vi "HOST Player Entry.vi"() -> ()   [LabVIEW 2026]
uses:
  Host State.ctl
  Leaderboard Announcement.ctl
  RT Commands.ctl
  RT Image.ctl
  Game Settings.ctl
  RT States.ctl
  Score.ctl
  SideSelector.ctl
  <vilib>/event_ctls.llb/eventvkey.ctl
  cee997e7-3729-4498-a080-51e98f020221.vi
  5b16e98e-8c62-4f4c-9228-1465c9ac843a.vi
  e3477a6d-3302-43e1-9f71-62fb47c8ca94.vi
  e2e9e0fd-3f68-41fd-9f22-0fd033314a53.vi
  <extravilib>/ChannelInstances/Tag-bool/Read With Abort.vi
  <extravilib>/ChannelInstances/Tag-bool/Write With Abort.vi
  <extravilib>/ChannelInstances/Tag-bool/Instantiate.vi
  <extravilib>/ChannelInstances/Tag-bool/EndpointRead.vi
  <extravilib>/ChannelInstances/Tag-bool/Endpoint.vi
  <extravilib>/ChannelInstances/Tag-bool.lvlib
panel:
  in  "path to PNG file":path
  in  "Button 1":bool
  in  "Player 1 Name":string
  in  "Button 2":bool
  in  "Player 2 Name":string
  in  "GO":bool
  out "error IO":errorcluster
  out "Status":string
  # "(ESC to abort round)"
  # "(Ctl+Shfit+GO! to terminate program)"
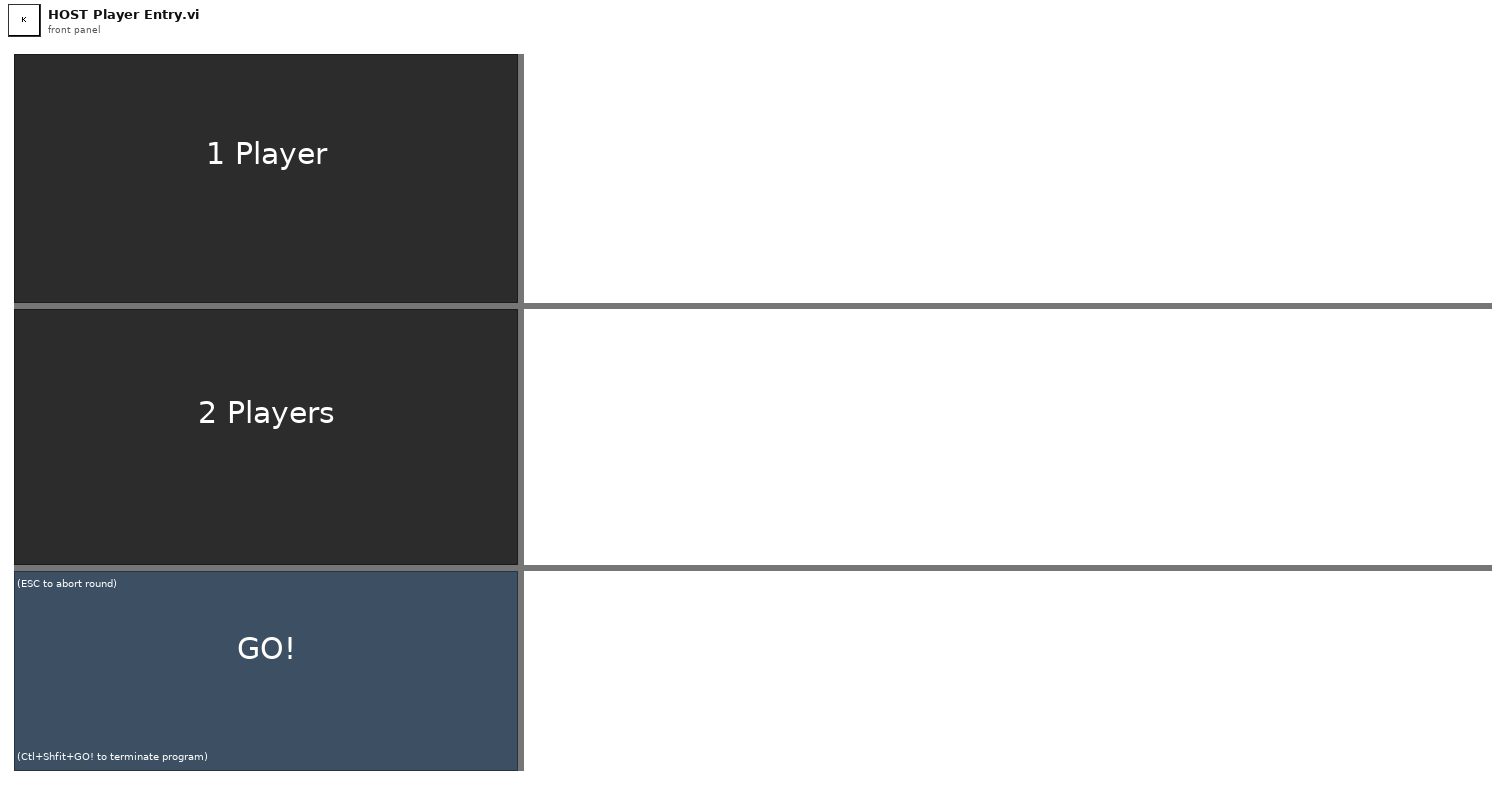
[diagram p1: front panel]
types:
  T1 = typedef "Leaderboard Announcement.ctl" = cluster{"Player 1 Name":string, "Score P1":u16, "Player 1 Name 2":string, "Score P1 2":u16}
  T2 = typedef "Host State.ctl" = enum16{"<startup>", "Idle", "StartGame", "WaitForCompletion", "Announce Winner"}
  T3 = typedef "RT Commands.ctl" = enum16{"<null>", "End Idle", "Reset", "Commit Settings", "Commit Host Settings"}
  T4 = typedef "Game Settings.ctl" = cluster{"Speed Threshold, ticks":u64, "Game Time":u32, "2 Players":bool}
  T5 = typedef "RT States.ctl" = enum16{"Idle", "Configuring", "1Player", "2Player", "Display Winner"}
  T6 = typedef "eventvkey.ctl" = enum16{"ASCII", "Enter", "Return", "Shift", "Ctrl", "Alt", "Cmd", "Opt", "Caps", "NumLock", "Clear", "Break", "Up", "Down", "Left", "Right", "Insert", "Delete", "Home", "End", "PageUp", "PageDown", "Escape", "Help", "Pause", "ScrollLock", "F1", "F2", "F3", "F4", "F5", "F6", "F7", "F8", "F9", "F10", "F11", "F12", "F13", "F14", "F15", "F16", "F17", "F18", "F19", "F20", "F21", "F22", "F23", "F24", "Play", "VolumeUp", "VolumeDown", "Mute", "Two Byte Char"}
  T7 = cluster{"left":i16, "top":i16, "right":i16, "bottom":i16}
  T8 = typedef "imagedata.ctl" = cluster{"image type":i32, "image depth":i32, "image":u8[], "mask":u8[], "colors":u32[], "Rectangle":cluster{"left":i16, "top":i16, "right":i16, "bottom":i16}}
  T9 = typedef "Score.ctl" = cluster{"Score P1":u16, "Score P2":u16, "Winner Selection":T10}
  T10 = typedef "SideSelector.ctl" = enum16{"P12", "P1", "P2"}
  T11 = cluster{"Player 1 Name":string, "Score P1":u16, "Player 2 Name":string, "Score P2":u16}
  T12 = typedef "Tag-bool.lvlib/))Channel.ctl" = refnum<queue>
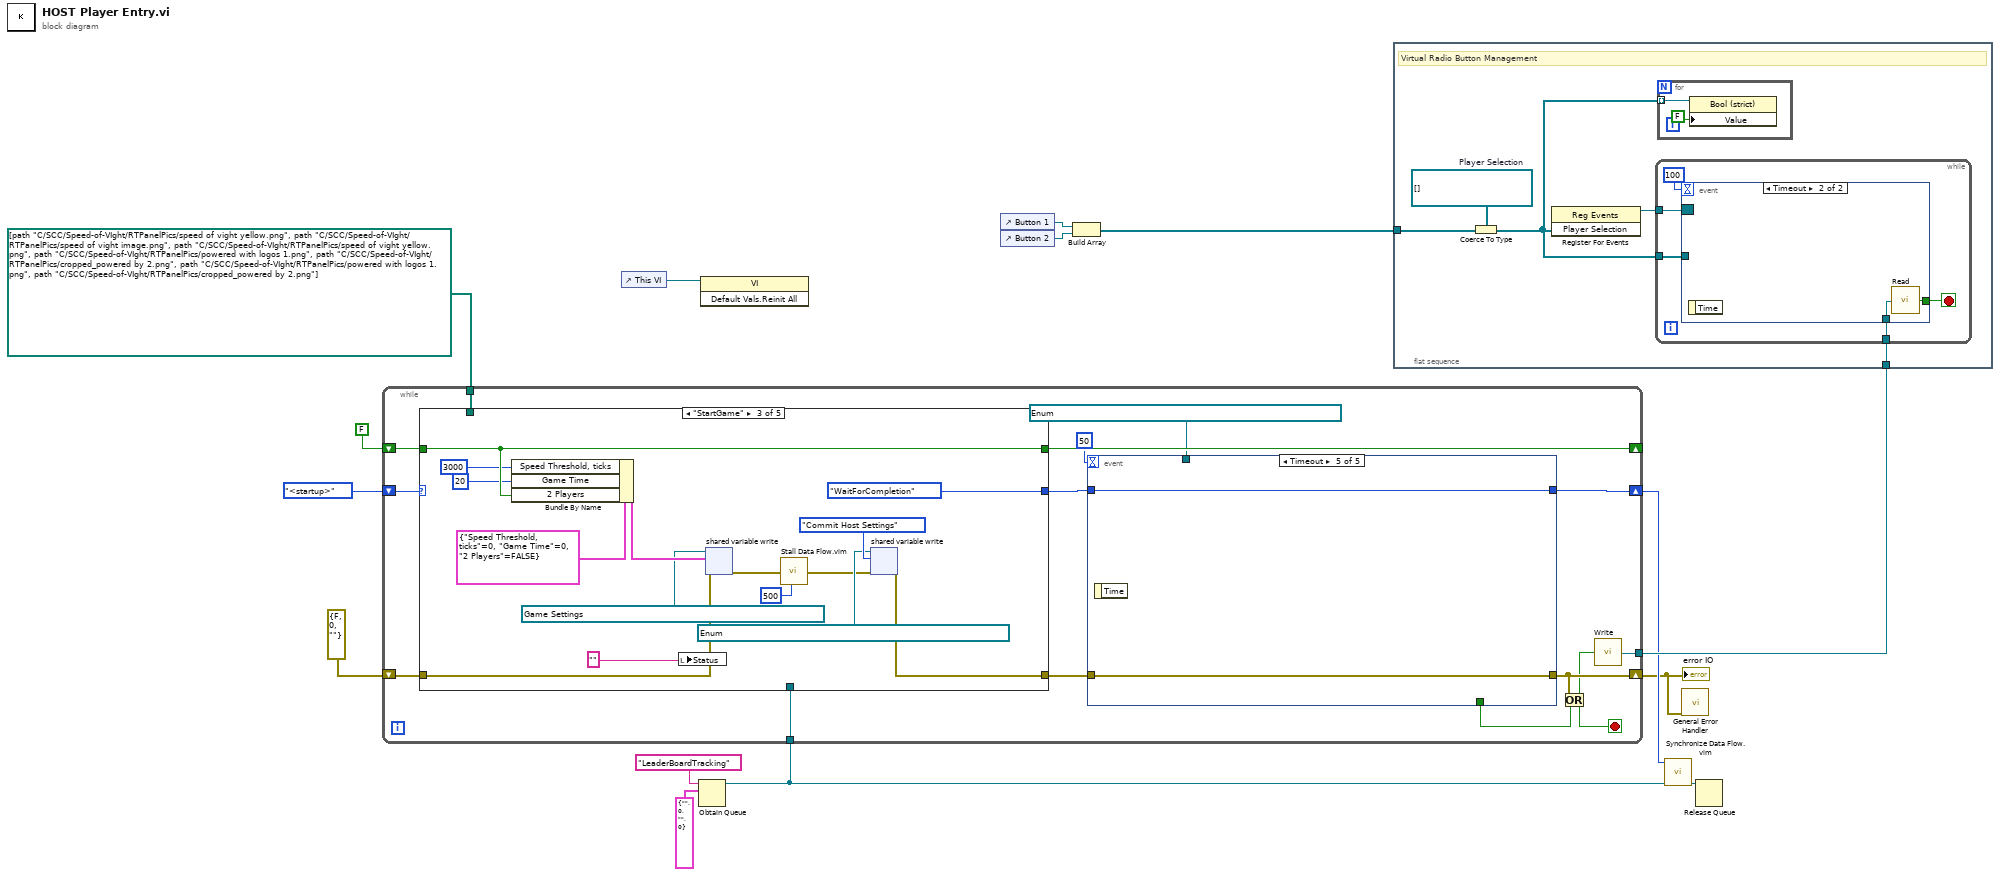
[diagram p0: block diagram]
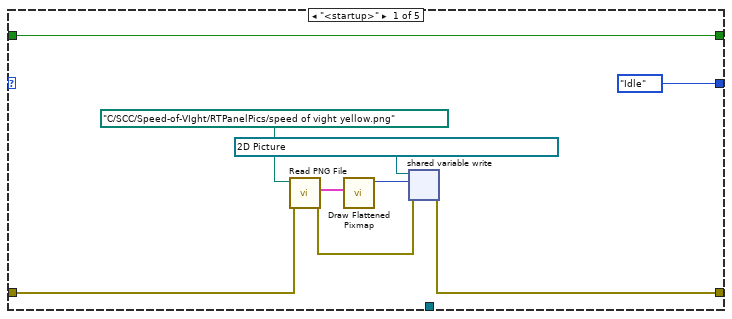
[diagram p2: hidden frame]
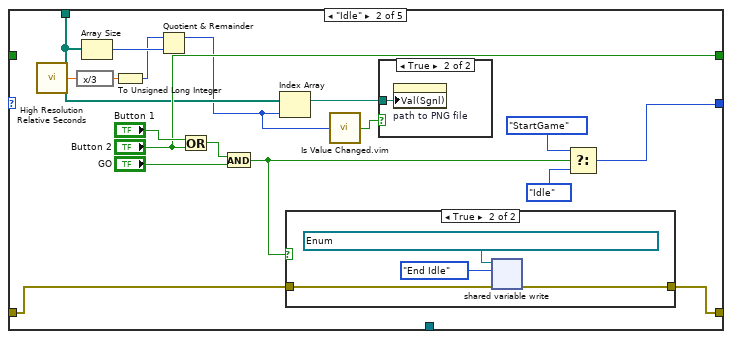
[diagram p3: hidden frame]
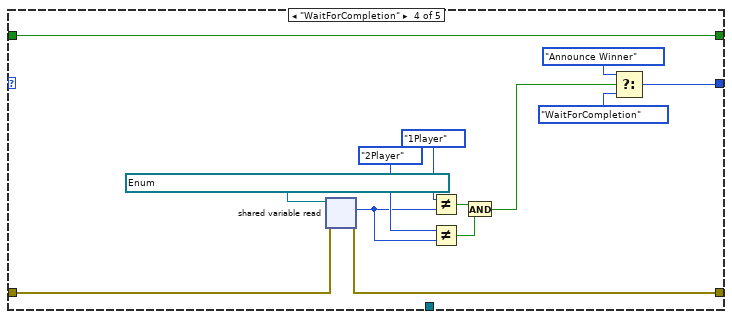
[diagram p6: hidden frame]
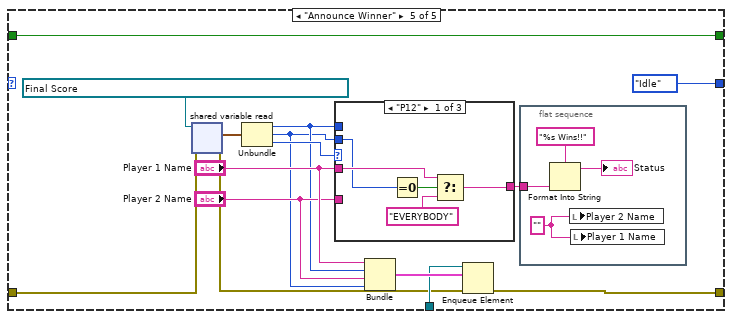
[diagram p7: hidden frame]
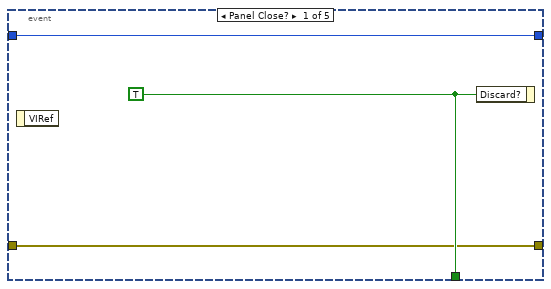
[diagram p10: hidden frame]
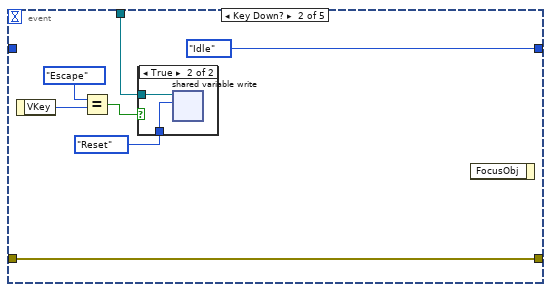
[diagram p11: hidden frame]
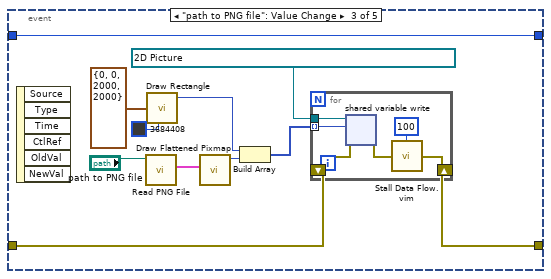
[diagram p13: hidden frame]
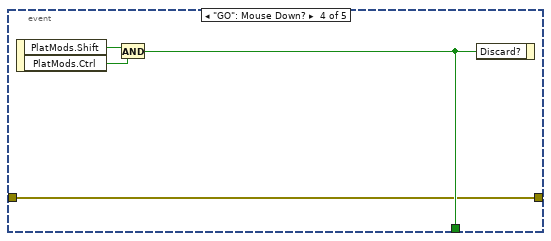
[diagram p14: hidden frame]
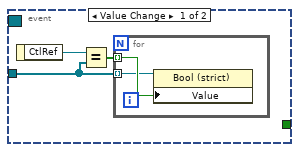
[diagram p15: hidden frame]
diagram:
  n1 = control-ref of="This VI"() -> (w10:refnum<vi>)
  n2 = Obtain Queue(name (unnamed)="LeaderBoardTracking", element data type=T1 {"Player 1 Name"="", "Score P1"=0, "Player 1 Name 2"="", "Score P1 2"=0} ("output cluster")) -> (queue out=w6:refnum<queue>)  [unwired: 3 in, 2 out]
  n3 = while {
    shift-right: [w26] -> w4
    shift-left: Host_State."<startup>" -> [w30]
    shift-right: [w29] -> _
    shift-left: FALSE ("Button 2") -> [w28]
    tunnel: [w24] -> w9
    tunnel: w6 -> [w23]
    shift-right: [w18] -> w1
    shift-left: errorcluster {"status"=FALSE, "code"=0, "source"=""} ("error IO") -> [w21]
    tunnel: path[] [path "C:/SCC/Speed-of-VIght/RTPanelPics/speed of vight yellow.png", path "C:/SCC/Speed-of-VIght/RTPanelPics/speed of vight image.png", path "C:/SCC/Speed-of-VIght/RTPanelPics/speed of vight yellow.png", path "C:/SCC/Speed-of-VIght/RTPanelPics/powered with logos 1.png", path "C:/SCC/Speed-of-VIght/RTPanelPics/cropped_powered by 2.png", path "C:/SCC/Speed-of-VIght/RTPanelPics/powered with logos 1.png", path "C:/SCC/Speed-of-VIght/RTPanelPics/cropped_powered by 2.png"] ("path to PNG file") -> [w19]
    stop <- w16 stop-if-true
    w22 = refnum<k21> "ni.var.psp://SpeedOfVIght/RT ShardVariables/H2RTCommand" items=["<null>", "End Idle", "Reset", "Commit Settings", "Commit Host Settings"] ("shared variable refnum in")
    n4 = case shown="\"StartGame\"" w30 {
      tunnel: [Host_State."Idle" w57 Host_State."WaitForCompletion" w88 Host_State."Idle" ("f")] -> w27
      tunnel: [w38 "Button 2" w75 w91 w105] -> w29
      tunnel: w28 -> [w38 _ w75 w91 w105]
      tunnel: w23 -> [_ _ _ _ w95]
      tunnel: [w32 w49 w64 w79 w92] -> w20
      tunnel: w21 -> [w31 w48 w65 w80 w94]
      tunnel: w19 -> [_ w46 _ _ _]
      frame "<startup>" {
        n5 = call <vilib>:"Read PNG File.vi"("error in (no error)"=w31, "path to PNG file"=path "C:/SCC/Speed-of-VIght/RTPanelPics/speed of vight yellow.png") -> ("error out"=w33:errorcluster, "image data"=w36:T8)  [unwired: 7 in, 1 out]
        n6 = call <vilib>:"Draw Flattened Pixmap.vi"("image data"=w36) -> ("new picture"=w37:picture)  [unwired: 8 in]
        n7 = shared-variable-write(refnum<k21> "ni.var.psp://SpeedOfVIght/RT ShardVariables/Idle Image" ("shared variable refnum in"), w33, w37) -> (w32:errorcluster)  [unwired: 1 out]
      }
      frame "Idle" {
        n8 = call <vilib>:"High Resolution Relative Seconds.vi"() -> ("relative seconds"=w44:dbl)
        n9 = expression code="x/3"(w44) -> (w43:dbl)
        n10 = Array Size(array=w46) -> (size(s)=w45:i32)
        n11 = To Unsigned Long Integer(number=w43) -> (unsigned 32bit integer=w42:u32)
        n12 = Quotient & Remainder(x=w42, y=w45) -> (x-y*floor(x/y)=w41:u32)  [unwired: 1 out]
        n13 = Or(x="Button 1", y="Button 2") -> (x .or. y?=w52:bool)
        n14 = And(x=w52, y="GO") -> (x .and. y?=w50:bool)
        n15 = Index Array(array=w46, index=w41) -> (element=w47:path)
        n16 = case shown="True" w50 {
          tunnel: [w59 w61] -> w49
          tunnel: w48 -> [w59 w60]
          frame False {
          }
          frame True {
            w63 = refnum<k21> "ni.var.psp://SpeedOfVIght/RT ShardVariables/H2RTCommand" items=["<null>", "End Idle", "Reset", "Commit Settings", "Commit Host Settings"] ("shared variable refnum in")
            n17 = shared-variable-write(w63, w60, RT_Commands."End Idle" ("H2RTCommand")) -> (w61:errorcluster)  [unwired: 1 out]
          }
        }
        n18 = call "Is Value Changed.vim"("value"=w41) -> ("changed or first call?"=w40:bool)
        n19 = case shown="True" w40 {
          tunnel: w47 -> [_ w58]
          frame False {
          }
          frame True {
            n20 = property on="path to PNG file" class="Path"("Val(Sgnl)"=w58) -> ()  [unwired: 2 in, 2 out]
          }
        }
        n21 = Select(t=Host_State."StartGame", s=w50, f=Host_State."Idle") -> (s? t:f=w57:T2)
      }
      frame "StartGame" {
        w70 = refnum<k21> "ni.var.psp://SpeedOfVIght/RT ShardVariables/H2RTCommand" items=["<null>", "End Idle", "Reset", "Commit Settings", "Commit Host Settings"] ("shared variable refnum in")
        n22 = Bundle By Name(cluster=T4 {"Speed Threshold, ticks"=0, "Game Time"=0, "2 Players"=FALSE} ("Game Settings"), "Speed Threshold, ticks"=u64 3000, "Game Time"=u32 20, "2 Players"=w75) -> (w76:T4)
        n23 = local write "Status"("" ("Player 2 Name")) -> ()
        n24 = shared-variable-write(refnum<k21> "ni.var.psp://SpeedOfVIght/RT ShardVariables/Game Settings" ("shared variable refnum in"), w65, w76) -> (w68:errorcluster)  [unwired: 1 out]
        n25 = call "Stall Data Flow.vim"("value in"=w68, "milliseconds to wait"=u32 500) -> ("value out"=w67:errorcluster)  [unwired: 1 out]
        n26 = shared-variable-write(w70, w67, RT_Commands."Commit Host Settings" ("H2RTCommand")) -> (w64:errorcluster)  [unwired: 1 out]
      }
      frame "WaitForCompletion" {
        w90 = refnum<k21> "ni.var.psp://SpeedOfVIght/RT ShardVariables/RT2HState" items=["Idle", "Configuring", "1Player", "2Player", "Display Winner"] ("shared variable refnum in")
        n27 = shared-variable-read(w90, w80) -> (w79:errorcluster, w83:T5)  [unwired: 1 out]
        n28 = Not Equal?(x=RT_States."1Player", y=w83) -> (x != y?=w87:bool)
        n29 = Not Equal?(x=RT_States."2Player", y=w83) -> (x != y?=w82:bool)
        n30 = And(x=w87, y=w82) -> (x .and. y?=w81:bool)
        n31 = Select(t=Host_State."Announce Winner", s=w81, f=Host_State."WaitForCompletion") -> (s? t:f=w88:T2)
      }
      frame "Announce Winner" {
        n32 = shared-variable-read(refnum<k21> "ni.var.psp://SpeedOfVIght/RT ShardVariables/Final Score" ("shared variable refnum in"), w94) -> (w93:errorcluster, w103:T9)  [unwired: 1 out]
        n33 = Unbundle(w103) -> ("Score P1"=w98:u16, "Score P2"=w97:u16, "Winner Selection"=w102:T10)
        n34 = case shown="\"P12\"" w102 {
          tunnel: [w113 w116 w117] -> w101
          tunnel: "Player 1 Name" -> [w112 w116 _]
          tunnel: "Player 2 Name" -> [_ _ w117]
          tunnel: w98 -> [_ _ _]
          tunnel: w97 -> [w111 _ _]
          frame "P12" {
            n35 = Equal To 0?(x=w111) -> (x = 0?=w115:bool)
            n36 = Select(t=w112, s=w115, f="EVERYBODY" ("Player 1 Name")) -> (s? t:f=w113:string)
          }
          frame "P1" {
          }
          frame "P2" {
          }
        }
        n37 = Bundle("Player 1 Name"="Player 1 Name", "Score P1"=w98, "Player 2 Name"="Player 2 Name", "Score P2"=w97) -> (w96:T11)  [unwired: 1 in]
        n38 = Enqueue Element(queue=w95, element=w96, error in (no error)=w93) -> (error out=w92:errorcluster)  [unwired: 1 in, 2 out]
        n39 = flat-sequence {
          tunnel: w101 -> [w108]
          frame #0 {
            w107 = "" ("Player 2 Name")
            n40 = Format Into String(format string="%s Wins!!", w108) -> (resulting string=→"Status":string)  [unwired: 2 in, 1 out]
            n41 = local write "Player 2 Name"(w107) -> ()
            n42 = local write "Player 1 Name"(w107) -> ()
          }
        }
      }
    }
    n43 = event shown="[4] Timeout" {
      selector: _ -> [_ _ _ _ _]
      dyn-events: _ -> [_ _ _ _ _]
      timeout: 50 -> [_ _ _ _ _]
      tunnel: w27 -> [w119 _ w135 _ w152]
      tunnel: [w120 _ _ w148 _] -> w17
      tunnel: [w119 Host_State."Idle" ("f") w135 _ w152] -> w26
      tunnel: w22 -> [_ w123 _ _ _]
      tunnel: w20 -> [w118 w121 w137 w147 w151]
      tunnel: [w118 w121 w136 w147 w151] -> w18
      event Panel Close? {
        w120 = TRUE ("Discard?")
        n44 = event-data() -> ()  [unwired: 1 in, 1 out]
        n45 = event-data("Discard?"=w120) -> ()  [unwired: 1 in, 1 out]
      }
      event Key Down? {
        n46 = event-data() -> ("VKey"=w127:T6)  [unwired: 1 in]
        n47 = Equal?(x=eventvkey."Escape" ("VKey"), y=w127) -> (x = y?=w125:bool)
        n48 = case shown="True" w125 {
          tunnel: w123 -> [_ w129]
          tunnel: RT_Commands."Reset" ("Enum") -> [_ w128]
          frame False {
          }
          frame True {
            n49 = shared-variable-write(w129, w128) -> ()  [unwired: 1 in, 2 out]
          }
        }
        n50 = event-data() -> ()  [unwired: 2 in, 1 out]
      }
      event "path to PNG file": Value Change {
        n51 = event-data() -> ()  [unwired: 1 in, 6 out]
        n52 = call <vilib>:"Read PNG File.vi"("path to PNG file"="path to PNG file") -> ("image data"=w138:T8)  [unwired: 8 in, 2 out]
        n53 = call <vilib>:"Draw Rectangle.vi"("rect"=T7 {"left"=0, "top"=0, "right"=2000, "bottom"=2000}, "color(black)"=u32 3684408) -> ("new picture"=w132:picture)  [unwired: 7 in]
        n54 = call <vilib>:"Draw Flattened Pixmap.vi"("image data"=w138) -> ("new picture"=w134:picture)  [unwired: 8 in]
        n55 = Build Array(w132, w134) -> (w133:picture[])
        n56 = for {
          tunnel: refnum<k21> "ni.var.psp://SpeedOfVIght/RT ShardVariables/Idle Image" ("shared variable refnum in") -> [w146]
          shift-right: [w142] -> w136
          shift-left: w137 -> [w145]
          tunnel: w133 -> [w143] mode=indexing
          n57 = shared-variable-write(w146, w145, w143) -> (w144:errorcluster)  [unwired: 1 out]
          n58 = call "Stall Data Flow.vim"("value in"=w144, "milliseconds to wait"=u32 100) -> ("value out"=w142:errorcluster)  [unwired: 1 out]
        }
      }
      event "GO": Mouse Down? {
        n59 = event-data() -> ("PlatMods.Shift"=w150:bool, "PlatMods.Ctrl"=w149:bool)  [unwired: 1 in]
        n60 = And(x=w150, y=w149) -> (x .and. y?=w148:bool)
        n61 = event-data("Discard?"=w148) -> ()  [unwired: 1 in, 1 out]
      }
      event Timeout {
        n62 = event-data() -> ()  [unwired: 1 in, 1 out]
      }
    }
    n63 = Or(x=w18, y=w17) -> (x .or. y?=w16:bool)
    n64 = call <extravilib>:"Write.vi"("element"=w16) -> ("channel"=w24:T12)  [unwired: 1 out]
  }
  "error IO" <- w1
  n65 = invoke class="VI" method="Default Vals.Reinit All"(reference=w10) -> ()  [unwired: 2 in, 3 out]
  n66 = control-ref of="Button 1"() -> (w15:refnum<vi>)
  n67 = control-ref of="Button 2"() -> (w14:refnum<vi>)
  n68 = Build Array(w15, w14) -> (w13:refnum<vi>[])
  n69 = flat-sequence {
    tunnel: w13 -> [w156]
    tunnel: w9 -> [w153]
    frame #0 {
      w154 = refnum<vi>[] []  # Player Selection
      # "Virtual Radio Button Management"
      n70 = Coerce To Type(0:w156, 1:w154) -> (2:w155:refnum<vi>[])
      n71 = register-events(w155) -> (reference out=w157:refnum<event-registration>)  [unwired: 2 in, 1 out]
      n72 = while {
        tunnel: w157 -> [w164]
        tunnel: w155 -> [w163]
        tunnel: w153 -> [w160]
        stop <- w162 stop-if-true
        n73 = event shown="[1] Timeout" {
          selector: w164 -> [_ _]
          dyn-events: _ -> [_ _]
          timeout: 100 -> [_ _]
          tunnel: w163 -> [w165 _]
          tunnel: [_ w170] -> w162
          tunnel: w160 -> [_ w171]
          event Value Change {
            n74 = event-data() -> ("CtlRef"=w167:refnum<vi>)  [unwired: 1 in]
            n75 = Equal?(x=w167, y=w165) -> (x = y?=w166:bool[])
            n76 = for {
              tunnel: w166 -> [w169] mode=indexing
              tunnel: w165 -> [w168] mode=indexing
              n77 = property class="Bool (strict)"(reference=w168, "Value"=w169) -> ()  [unwired: 1 in, 2 out]
            }
          }
          event Timeout {
            n78 = event-data() -> ()  [unwired: 1 in, 1 out]
            n79 = call <extravilib>:"Read.vi"("channel"=w171) -> ("element"=w170:bool)  [unwired: 1 in, 1 out]
          }
        }
      }
      n80 = for {
        tunnel: w155 -> [w159] mode=indexing
        n81 = property class="Bool (strict)"(reference=w159, "Value"=FALSE) -> ()  [unwired: 1 in, 2 out]
      }
    }
  }
  n82 = call "Synchronize Data Flow.vim"("input 4"=w6, "input 1"=w4) -> ("output 4"=w5:refnum<queue>)  [unwired: 2 in, 3 out]
  n83 = call <vilib>:"General Error Handler.vi"("error in (no error)"=w1) -> ()  [unwired: 10 in, 5 out]
  n84 = Release Queue(queue=w5) -> ()  [unwired: 2 in, 3 out]
